vi "torsional-error-handler.vi"(1 "error in":errorcluster) -> ()   [LabVIEW 2013]
panel:
  # "This is a specialized error handler.  It shows known-work arounds for particular errors, or uses the simple error handler for all others."
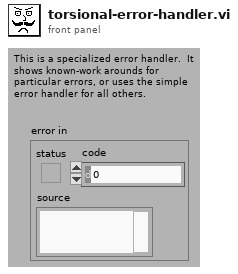
[diagram p1: front panel]
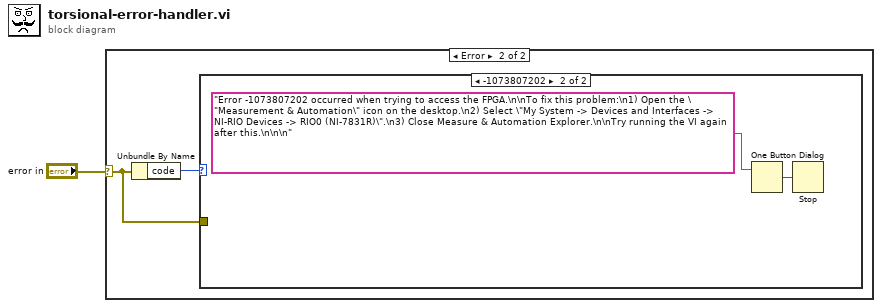
[diagram p0: block diagram]
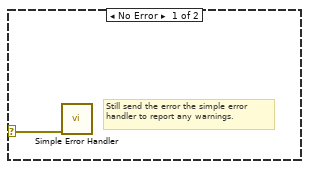
[diagram p2: hidden frame]
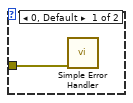
[diagram p3: hidden frame]
diagram:
  n1 = case shown="Error" "error in" {
    selector: "error in" -> [w2 w3]
    frame No Error {
      # "Still send the error the simple error handler to report any warnings."
      n2 = call <vilib>:"Simple Error Handler.vi"("error in (no error)"=w2) -> ()  [unwired: 4 in, 5 out]
    }
    frame Error {
      n3 = Unbundle By Name(w3) -> ("code"=w4:i32)
      n4 = case shown="-1073807202" w4 {
        tunnel: w3 -> [w5 _]
        frame 0, Default {
          n5 = call <vilib>:"Simple Error Handler.vi"("error in (no error)"=w5) -> ()  [unwired: 4 in, 5 out]
        }
        frame -1073807202 {
          n6 = One Button Dialog(message="Error -1073807202 occurred when trying to access the FPGA.\n\nTo fix this problem:\n1) Open the \"Measurement & Automation\" icon on the desktop.\n2) Select \"My System -> Devices and Interfaces -> NI-RIO Devices -> RIO0 (NI-7831R)\".\n3) Close Measure & Automation Explorer.\n\nTry running the VI again after this.\n\n\n") -> (true=w7:bool)  [unwired: 1 in]
          n7 = Stop(stop? (T)=w7) -> ()
        }
      }
    }
  }
